vi "Drive_Globals.vi"() -> ()   [LabVIEW 2019]
uses:
  Subsystems/Drive/DriveExecuteCluster.ctl
  Subsystems/Drive/DriveSetCluster.ctl
panel:
  in  "Drive Set Notifier":refnum<notifier>
  in  "Drive Execute Notifier":refnum<notifier>
  in  "Drive Set Refnum":string="Drive Set"
  in  "Drive Execute Refnum":string="Drive Execute"
  in  "Left Master Refnum":string="Left Master"
  in  "Left Slave Refnum":string="Left Slave"
  in  "Right Slave Refnum":string="Right Slave"
  in  "Right Master Refnum":string="Right Master"
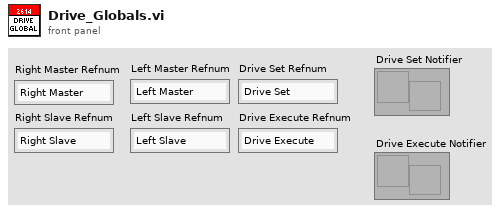
[diagram p1: front panel]
diagram:
